vi "Init.vi"(8 "error in (no error)":errorcluster, 10 "Waveform Settings":T1, 11 "Waveform Generator in":refnum<class "Waveform Generator.lvclass">) -> (0 "error out":errorcluster, 3 "Waveform Generator out":refnum<class "Waveform Generator.lvclass">)   [LabVIEW 2015, in "Waveform Generator.lvclass"]
uses:
  Waveform Generator.lvclass
  Typedefs/Waveform Settings.ctl
  Typedefs/Waveform Types.ctl
  Waveform Generator.lvclass/Waveform Generator.ctl
  Typedefs/FAMT Typedefs.lvlib
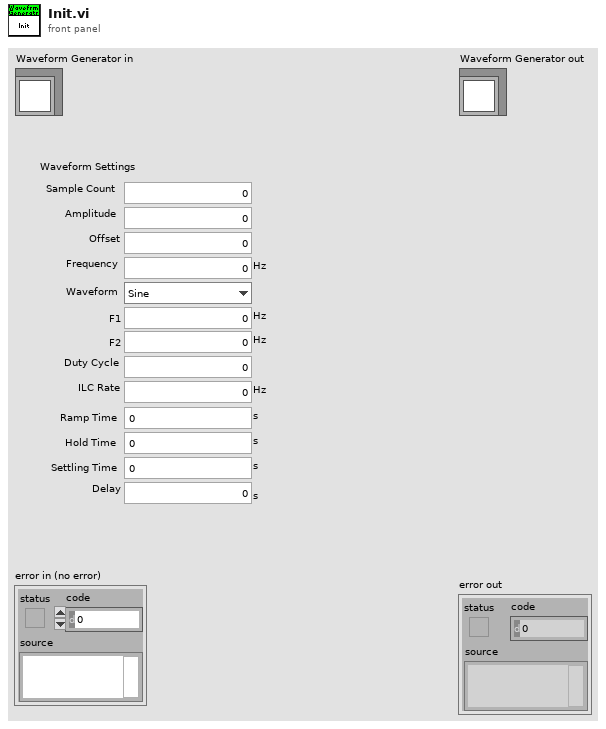
[diagram p1: front panel]
types:
  T1 = typedef "FAMT Typedefs.lvlib/Waveform Settings.ctl" = cluster{"Sample Count":u32, "Amplitude":dbl, "Offset":dbl, "Frequency":dbl[unit], "Waveform":T2, "F1":dbl[unit], "F2":dbl[unit], "Duty Cycle":dbl, "ILC Rate":dbl[unit], "Ramp Time":dbl[unit], "Hold Time":dbl[unit], "Settling Time":dbl[unit], "Delay":dbl[unit]}
  T2 = typedef "FAMT Typedefs.lvlib/Waveform Types.ctl" = enum16{"Sine", "Triangle", "Square", "Sawtooth", "Chirp", "Gaussian", "Trapezoid"}
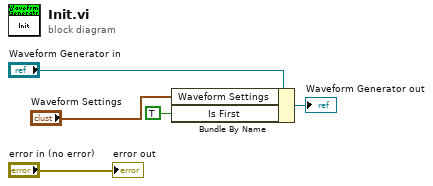
[diagram p0: block diagram]
diagram:
  n1 = Bundle By Name(cluster="Waveform Generator in", "Waveform Settings"="Waveform Settings", "Is First"=TRUE ("IsFirst")) -> (→"Waveform Generator out":refnum<class "Waveform Generator.lvclass">)
  "error out" <- "error in (no error)"
